vi "Plot_Channels_Sub.vi"(4 "End Time":dbl, 5 "precision":string, 7 "Mode":T1(ring), 8 "History (min)":dbl format="%.1f", 9 "Search String":string, 10 "Selector List In":string[](array[string]), 11 "Selector array In":i32[](array[numeric])) -> (0 "Plot Legend":string[](array[string]), 1 "Plot":cluster{"Times":dbl[], "Output array":dbl[]}[](graph), 2 "Selector List Out":string[](array[string]), 3 "Selector array Out":i32[](array[numeric]), 6 "Selector Changed?":bool)   [LabVIEW 2010]
uses:
  ADAM Controls/Search_mode.ctl
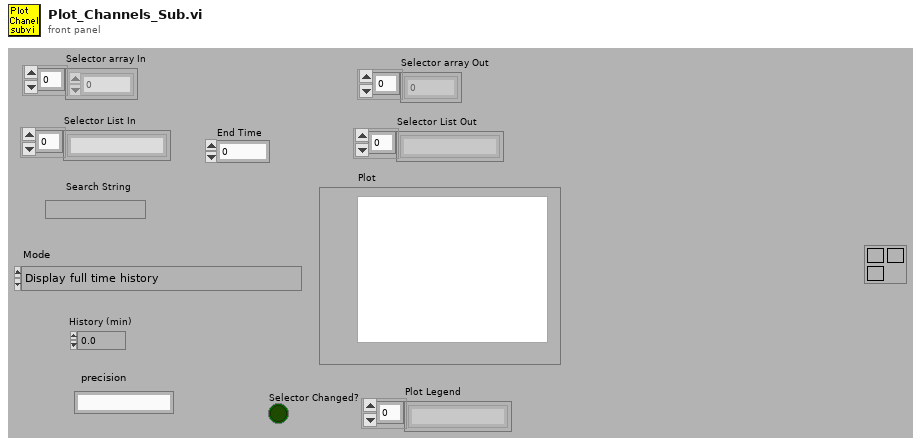
[diagram p1: front panel]
types:
  T1 = enum16{"Display full time history", "Display data over specified period"}
  T2 = typedef "Search_mode.ctl" = enum16{"Between times", "All Times"}
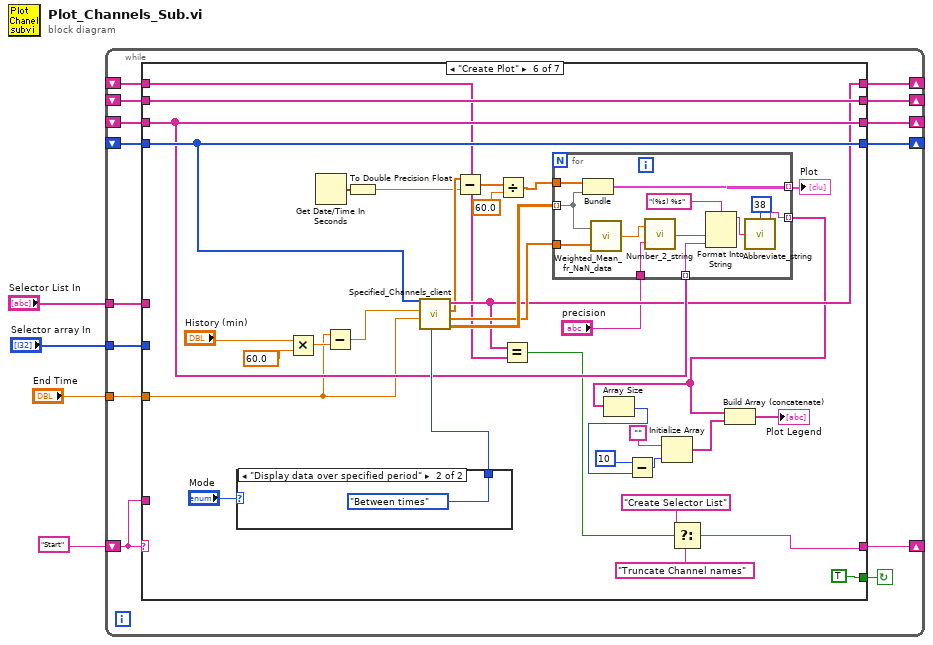
[diagram p0: block diagram]
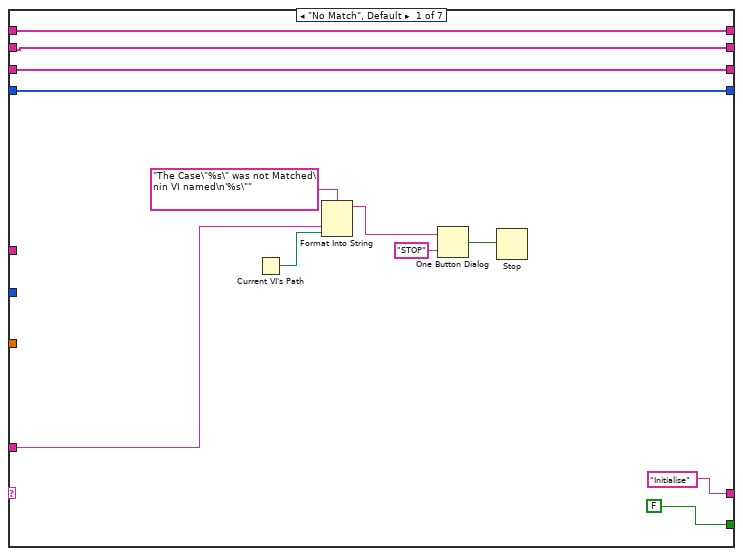
[diagram p2: hidden frame]
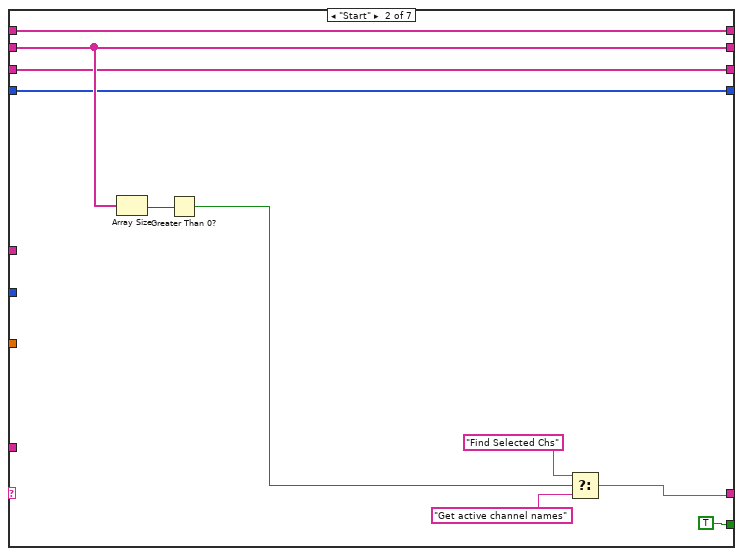
[diagram p3: hidden frame]
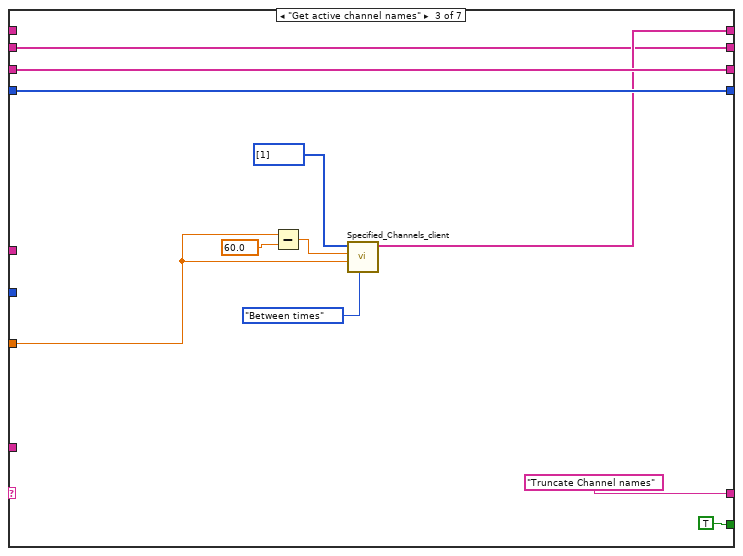
[diagram p4: hidden frame]
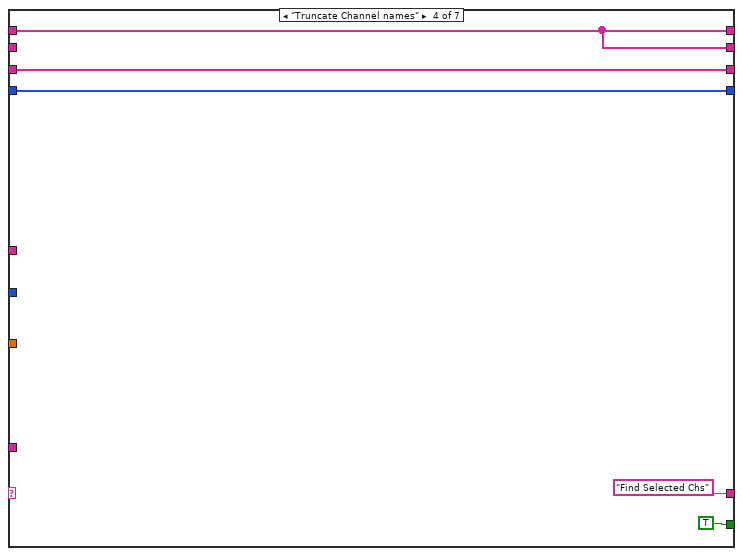
[diagram p5: hidden frame]
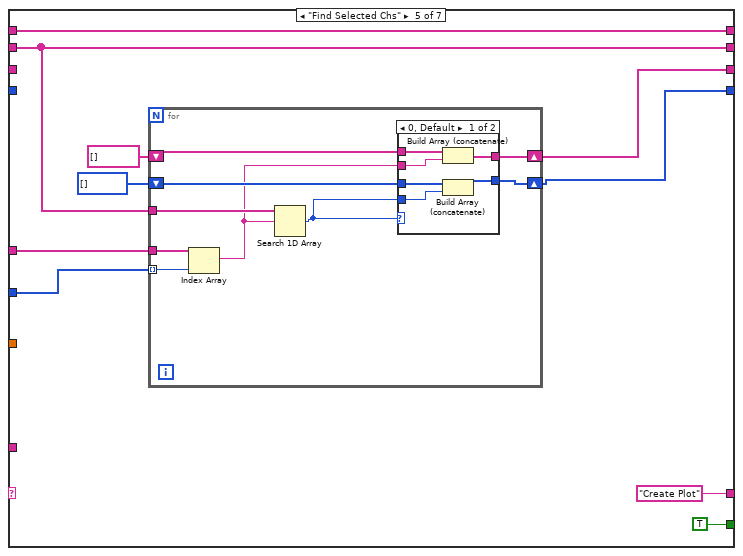
[diagram p6: hidden frame]
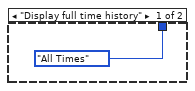
[diagram p8: hidden frame]
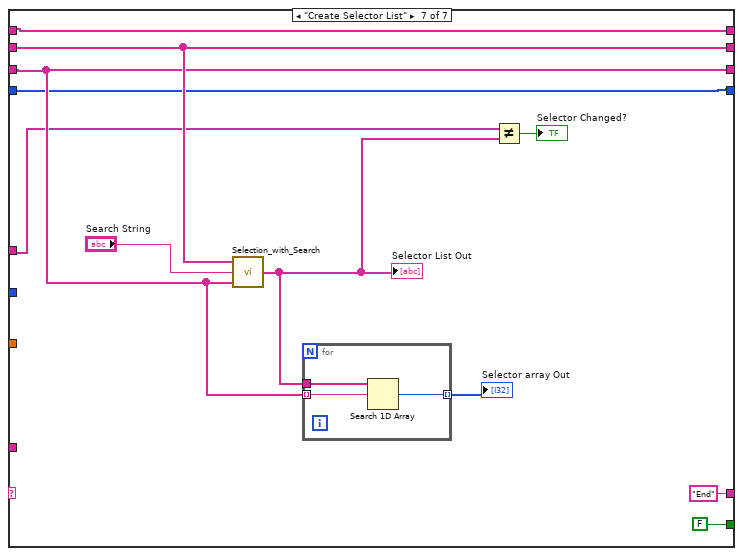
[diagram p9: hidden frame]
diagram:
  n1 = while {
    shift-left: "Start" -> [w16]
    shift-right: [w17] -> _
    shift-right: [w13] -> _
    shift-left: _ -> [w15]
    tunnel: "End Time" -> [w14]
    tunnel: "Selector List In" -> [w12]
    tunnel: "Selector array In" -> [w11]
    shift-right: [w10] -> _
    shift-left: _ -> [w7]
    shift-right: [w9] -> _
    shift-left: _ -> [w8]
    shift-right: [w6] -> _
    shift-left: _ -> [w5]
    stop <- w18 continue-if-true
    n2 = case shown="\"Create Plot\"" w16 {
      tunnel: [FALSE TRUE TRUE TRUE TRUE TRUE FALSE] -> w18
      tunnel: ["Initialise" w35 "Truncate Channel names" "Find Selected Chs" "Create Plot" w99 "End"] -> w17
      tunnel: w16 -> [w25 _ _ _ _ _ _]
      tunnel: w15 -> [w22 w34 w41 _ w62 w105 w141]
      tunnel: w14 -> [_ _ w49 _ _ w96 _]
      tunnel: [w22 w34 w41 w52 w62 w105 w141] -> w13
      tunnel: w12 -> [_ _ _ _ w65 _ w133]
      tunnel: w11 -> [_ _ _ _ w64 _ _]
      tunnel: [w21 w33 w44 w54 w61 w106 w139] -> w10
      tunnel: [w20 w32 w43 w53 w60 w107 w138] -> w9
      tunnel: w8 -> [w20 w32 w43 w53 _ w107 w138]
      tunnel: w7 -> [w21 w33 w44 w54 _ w106 w139]
      tunnel: [w19 w31 w42 w52 w57 w104 w135] -> w6
      tunnel: w5 -> [w19 w31 _ w52 w57 w103 w135]
      frame "No Match", Default {
        n3 = Current VI's Path() -> (path=w24:path)
        n4 = Format Into String(format string="The Case\"%s\" was not Matched\nin VI named\n'%s\"" ("Format String"), w25, w24) -> (resulting string=w28:string)  [unwired: 2 in, 1 out]
        n5 = One Button Dialog(message=w28, button name ("OK")="STOP") -> (true=w26:bool)
        n6 = Stop(stop? (T)=w26) -> ()
      }
      frame "Start" {
        n7 = Array Size(array=w34) -> (size(s)=w39:i32)
        n8 = Greater Than 0?(x=w39) -> (x > 0?=w38:bool)
        n9 = Select(t="Find Selected Chs", s=w38, f="Get active channel names") -> (s? t:f=w35:string)
      }
      frame "Get active channel names" {
        n10 = Subtract(x=w49, y=60.0) -> (x-y=w47:dbl)
        n11 = call "Specified_Channels_client.vi"("Mode"=Search_mode."Between times", "End time"=w49, "Start time"=w47, "ADAM Index array"=i32[] [1]) -> ("All Active Ch Names"=w42:string[])  [unwired: 1 in, 6 out]
      }
      frame "Truncate Channel names" {
      }
      frame "Find Selected Chs" {
        n12 = for {
          tunnel: w62 -> [w75]
          shift-right: [w73] -> w60
          shift-left: i32[] [] -> [w74]
          shift-right: [w68] -> w61
          shift-left: string[] [] -> [w69]
          tunnel: w65 -> [w71]
          tunnel: w64 -> [w70] mode=indexing
          n13 = Index Array(array=w71, index=w70) -> (element=w67:string)
          n14 = Search 1D Array(1D array=w75, element=w67) -> (index of element=w72:i32)  [unwired: 1 out]
          n15 = case shown="0, Default" w72 {
            tunnel: w74 -> [w81 w83]
            tunnel: [w80 w83] -> w73
            tunnel: w72 -> [w79 _]
            tunnel: w69 -> [w78 w82]
            tunnel: [w77 w82] -> w68
            tunnel: w67 -> [w76 _]
            frame 0, Default {
              n16 = Build Array (concatenate)(w78, w76) -> (w77:string[])
              n17 = Build Array (concatenate)(w81, w79) -> (w80:i32[])
            }
            frame -1 {
            }
          }
        }
      }
      frame "Create Plot" {
        n18 = case shown="\"Display data over specified period\"" "Mode" {
          tunnel: [Search_mode."All Times" ("Mode") Search_mode."Between times" ("Mode")] -> w108
          frame "Display full time history" {
          }
          frame "Display data over specified period" {
          }
        }
        n19 = Multiply(x="History (min)", y=60.0) -> (x*y=w115:dbl)
        n20 = Get Date/Time In Seconds() -> (seconds since 1Jan1904=w85:timestamp)
        n21 = Subtract(x=w96, y=w115) -> (x-y=w112:dbl)
        n22 = To Double Precision Float(number=w85) -> (double precision float=w84:dbl)
        n23 = call "Specified_Channels_client.vi"("Mode"=w108, "End time"=w96, "Start time"=w112, "ADAM Index array"=w107) -> ("Output array"=w111:dbl[][], "Averaging Period"=w109:dbl[], "Centre Times"=w95:dbl[], "All Active Ch Names"=w104:string[])  [unwired: 1 in, 3 out]
        n24 = Subtract(x=w95, y=w84) -> (x-y=w98:dbl[])
        n25 = Divide(x=w98, y=60.0) -> (x/y=w94:dbl[])
        n26 = Equal?(x=w104, y=w103) -> (x = y?=w102:bool)
        n27 = for {
          tunnel: w111 -> [w128] mode=indexing
          tunnel: [w129] -> w110 mode=indexing
          tunnel: w94 -> [w127]
          tunnel: w109 -> [w126]
          tunnel: w106 -> [w125] mode=indexing
          tunnel: [w121] -> w90 mode=indexing
          tunnel: "precision" -> [w118]
          n28 = Bundle(w127, "Output array"=w128) -> (w129:cluster{dbl[], "Output array":dbl[]})  [unwired: 1 out]
          n29 = call "Weighted_Mean_fr_NaN_data.vi"("Weighting"=w126, "Data"=w128) -> ("Mean value"=w120:dbl)
          n30 = call "Number_2_string.vi"("precision"=w118, "number"=w120) -> ("String"=w119:string)
          n31 = Format Into String(format string="(%s) %s", w119, w125) -> (resulting string=w122:string)  [unwired: 2 in, 1 out]
          n32 = call "Abbreviate_string.vi"("Input String"=w122, "Max String Length"=38) -> ("Output String"=w121:string)
        }
        "Plot" <- w110
        n33 = Array Size(array=w90) -> (size(s)=w88:i32)
        n34 = Subtract(x=10 ("dimension size"), y=w88) -> (x-y=w87:i32)
        n35 = Initialize Array("", w87) -> (w91:string[])
        n36 = Select(t="Create Selector List", s=w102, f="Truncate Channel names") -> (s? t:f=w99:string)
        n37 = Build Array (concatenate)(w90, w91) -> (→"Plot Legend":string[])
      }
      frame "Create Selector List" {
        n38 = call "Selection_with_Search.vi"("Selected Channel Names"=w139, "Search String"="Search String", "All Channel Names"=w141) -> ("Item Names"=w134:string[])
        "Selector List Out" <- w134
        n39 = for {
          tunnel: w134 -> [w145]
          tunnel: w139 -> [w144] mode=indexing
          tunnel: [w143] -> w140 mode=indexing
          n40 = Search 1D Array(1D array=w145, element=w144) -> (index of element=w143:i32)  [unwired: 1 out]
        }
        "Selector array Out" <- w140
        n41 = Not Equal?(x=w133, y=w134) -> (x != y?=→"Selector Changed?":bool)
      }
    }
  }
